vi "path file filter.vi"(8 "Sys Error In":errorcluster, 10 "file type":string="*.txt", 11 "path":path) -> (0 "错误输出":errorcluster, 3 "File path":path)   [LabVIEW 2018]
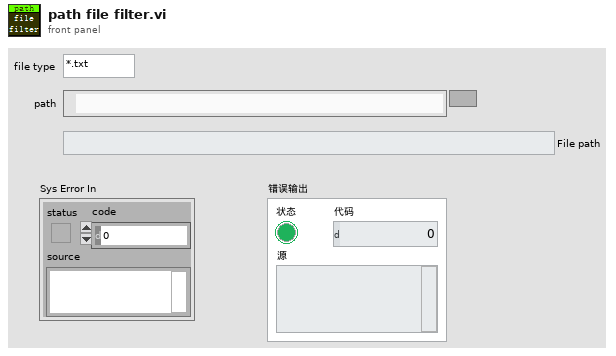
[diagram p1: front panel]
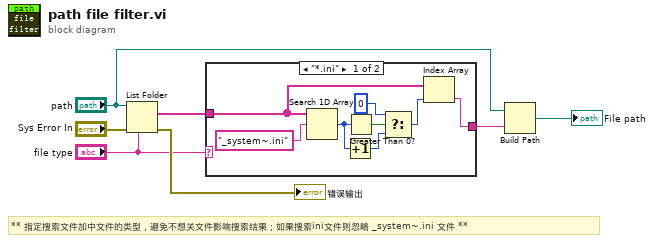
[diagram p0: block diagram]
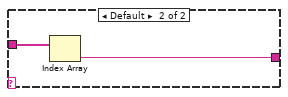
[diagram p2: hidden frame]
diagram:
  # "** 指定搜索文件加中文件的类型，避免不想关文件影响搜索结果；如果搜索ini文件则忽略 _system~.ini 文件 **"
  n1 = List Folder(path="path", pattern="file type", error in="Sys Error In") -> (filenames=w6:string[], error out=→"错误输出":errorcluster)  [unwired: 1 in, 2 out]
  n2 = case shown="\"*.ini\"" "file type" {
    tunnel: w6 -> [w10 w17]
    tunnel: [w8 w16] -> w4
    frame "*.ini" {
      n3 = Search 1D Array(1D array=w10, element="_system~.ini") -> (index of element=w12:i32)  [unwired: 1 in]
      n4 = Increment(x=w12) -> (x+1=w11:i32)
      n5 = Greater Than 0?(x=w12) -> (x > 0?=w14:bool)
      n6 = Select(t=u8 0, s=w14, f=w11) -> (s? t:f=w9:i32)
      n7 = Index Array(array=w10, index=w9) -> (element=w8:string)
    }
    frame Default {
      n8 = Index Array(array=w17) -> (element=w16:string)  [unwired: 1 in]
    }
  }
  n9 = Build Path(base path="path", name or relative path=w4) -> (appended path=→"File path":path)
